vi "Define_dR_Area_for_101_Displ-1.vi"(4 "[IN] Areas particles\nPrimary Detected":dbl[][](array[numeric]), 6 "[IN] Primary \n(X,Y) Detected":dbl[][](array[numeric]), 8 "error IN":errorcluster, 9 "[IN] Subtrack":T1, 11 "[IN] Still connect\ned tracks in group":T2) -> (0 "error OUT":errorcluster, 2 "[OUT] Area of  \"101\" \ndestination point":dbl, 3 "[OUT] dR for 101 \ndisplacement":dbl)   [LabVIEW 2013]
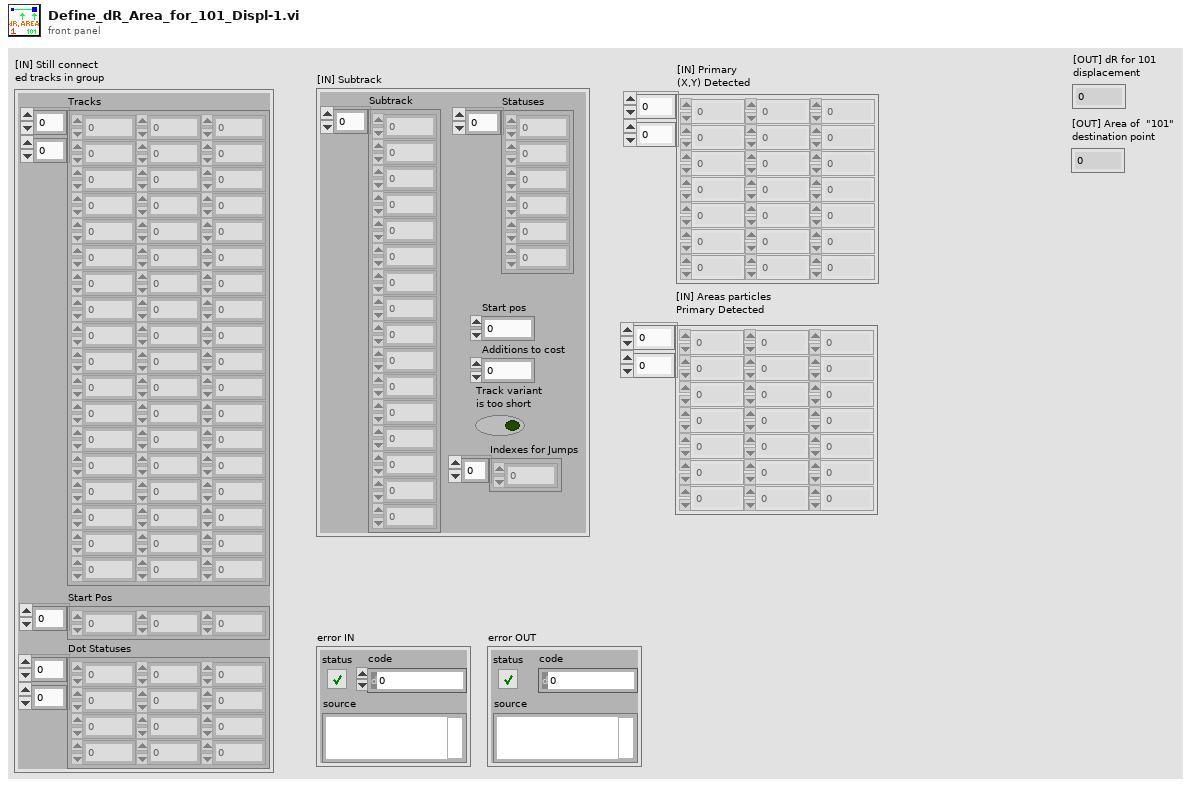
[diagram p1: front panel]
types:
  T1 = cluster{"Subtrack":dbl[], "Statuses":i16[], "Start pos":i32, "Additions to cost":i32, "Track variant \nis too short":bool, "Indexes for Jumps":i32[]}
  T2 = cluster{"Tracks":dbl[][], "Start Pos":i32[], "Dot Statuses":i16[][]}
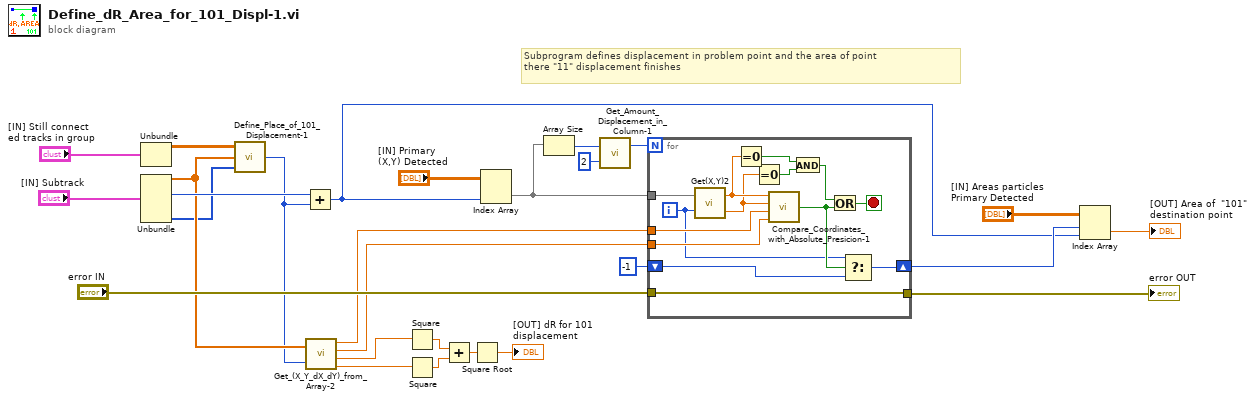
[diagram p0: block diagram]
diagram:
  # "Subprogram defines displacement in problem point and the area of point \nthere \"11\" displacement finishes"
  n1 = Unbundle("[IN] Still connect\ned tracks in group") -> ("Tracks"=w4:dbl[][])  [unwired: 2 out]
  n2 = Unbundle("[IN] Subtrack") -> ("Subtrack"=w3:dbl[], "Start pos"=w16:i32, "Indexes for Jumps"=w2:i32[])  [unwired: 3 out]
  n3 = call "Define_Place_of_101_Displacement-1.vi"("[IN] Indexes for Jumps"=w2, "[IN] Subtrack"=w3, "[IN] Tracks"=w4) -> ("[OUT] Index of \"11\" Dis\nplacement in Subtrack"=w1:i32)  [unwired: 2 in]
  n4 = Add(x=w16, y=w1) -> (x+y=w7:i32)
  n5 = call "Get_(X_Y_dX_dY)_from_Array-2.vi"("(X,Y,dX,dY)"=w3, "Index of Displacement"=w1) -> ("X"=w5:dbl, "Y"=w6:dbl, "dX"=w9:dbl, "dY"=w8:dbl)
  n6 = Square(x=w9) -> (x^2=w25:dbl)
  n7 = Square(x=w8) -> (x^2=w24:dbl)
  n8 = Add(x=w25, y=w24) -> (x+y=w23:dbl)
  n9 = Square Root(x=w23) -> (sqrt(x)=→"[OUT] dR for 101 \ndisplacement":dbl)
  n10 = Index Array(array="[IN] Primary \n(X,Y) Detected", index (col)=w7) -> (element=w17:dbl[])  [unwired: 1 in]
  n11 = Array Size(array=w17) -> (size(s)=w21:i32)
  n12 = call "Get_Amount_Displacement_in_Column-1.vi"("multiplier"=2, "# Rows"=w21) -> ("Displ amount"=w19:i32)  [unwired: 1 out]
  n13 = for {
    N: w19 -> [_]
    tunnel: w17 -> [w40]
    tunnel: w5 -> [w39]
    tunnel: w6 -> [w38]
    shift-right: [w29] -> w11
    shift-left: -1 -> [w30]
    tunnel: "error IN" -> [w28]
    tunnel: [w28] -> w13
    i -> [w31]
    stop <- w41 stop-if-true
    n14 = call "Get(X,Y)2.vi"("[IN] index of (X,Y)"=w31, "[IN] Array coordi\nnates (X,Y) in Frame"=w40) -> ("[OUT] Y"=w34:dbl, "[OUT] X"=w35:dbl)
    n15 = Equal To 0?(x=w35) -> (x = 0?=w37:bool)
    n16 = Equal To 0?(x=w34) -> (x = 0?=w36:bool)
    n17 = call "Compare_Coordinates_with_Absolute_Presicion-1.vi"("X 1"=w35, "Y 1"=w34, "X 2"=w39, "Y 2"=w38) -> ("[OUT] Same coordinates?"=w32:bool)  [unwired: 1 in]
    n18 = And(x=w37, y=w36) -> (x .and. y?=w33:bool)
    n19 = Or(x=w33, y=w32) -> (x .or. y?=w41:bool)
    n20 = Select(t=w31, s=w32, f=w30) -> (s? t:f=w29:i32)
  }
  "error OUT" <- w13
  n21 = Index Array(array="[IN] Areas particles\nPrimary Detected", index (row)=w11, index (col)=w7) -> (element=→"[OUT] Area of  \"101\" \ndestination point":dbl)
